vi "TWM Client Cmd Set Measurement.vi"(6 "Trigger":T1, 7 "end of packet key":string="TWM:command:EndOfPacket", 8 "error in":errorcluster, 9 "processing":T2, 10 "meas":T3, 11 "handle":i32) -> (0 "error out":errorcluster, 3 "handle out":i32)   [LabVIEW 2020, in "TWM Client.lvlib"]
doc: "Write Set measurement command packet to TWM server. Sets measurement configuration and processing configuration. The item \"valid?\" of the cluster(s) must be set to \"True\" to send the setup."
uses:
  TWM Client.lvlib
  TWM Client Meas Setup.ctl
  TWM Client Processing Setup.ctl
  TWM Client Meas Setup Trig.ctl
  I64.vi
  EXT.vi
  1D EXT.vi
  String.vi
  1D String.vi
  infolib.lvlib
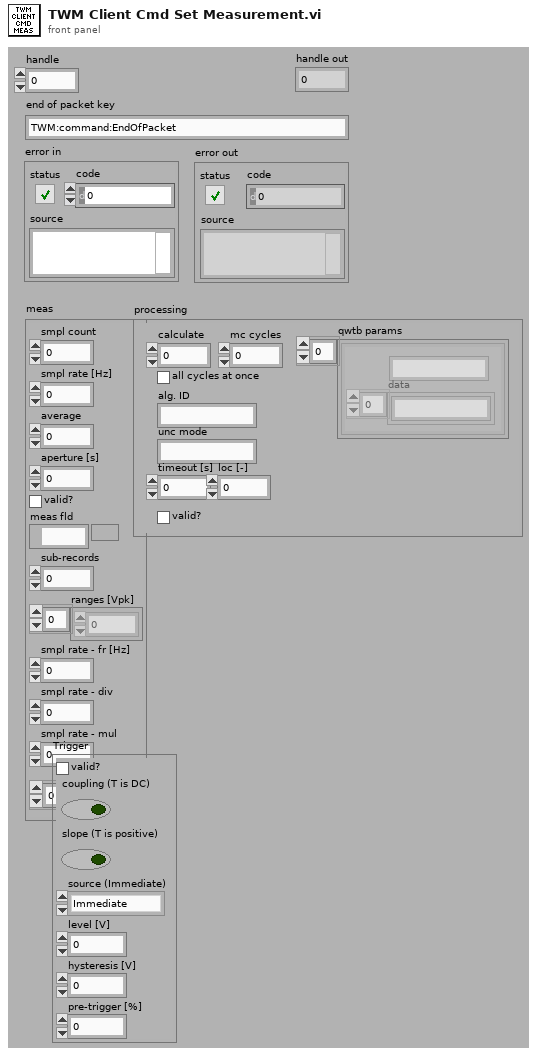
[diagram p1: front panel]
types:
  T1 = typedef "TWM Client.lvlib/TWM Client Meas Setup Trig.ctl" = cluster{"valid?":bool, "coupling (T is DC)":bool, "slope (T is positive)":bool, "source (Immediate)":enum16{"Immediate", "Level", "External"}, "level [V]":dbl, "hysteresis [V]":dbl, "pre-trigger [%]":dbl}
  T2 = typedef "TWM Client.lvlib/TWM Client Processing Setup.ctl" = cluster{"calculate":i32, "all cycles at once":bool, "alg. ID":string, "unc mode":string, "mc cycles":i32, "timeout [s]":dbl, "loc [-]":dbl, "valid?":bool, "qwtb params":cluster{"name":string, "data":string[]}[]}
  T3 = typedef "TWM Client.lvlib/TWM Client Meas Setup.ctl" = cluster{"smpl count":i32, "smpl rate [Hz]":dbl, "average":i32, "aperture [s]":dbl, "valid?":bool, "meas fld":path, "sub-records":i32, "ranges [Vpk]":dbl[], "smpl rate - fr [Hz]":dbl, "smpl rate - div":dbl, "smpl rate - mul":dbl, "offsets [V]":dbl[]}
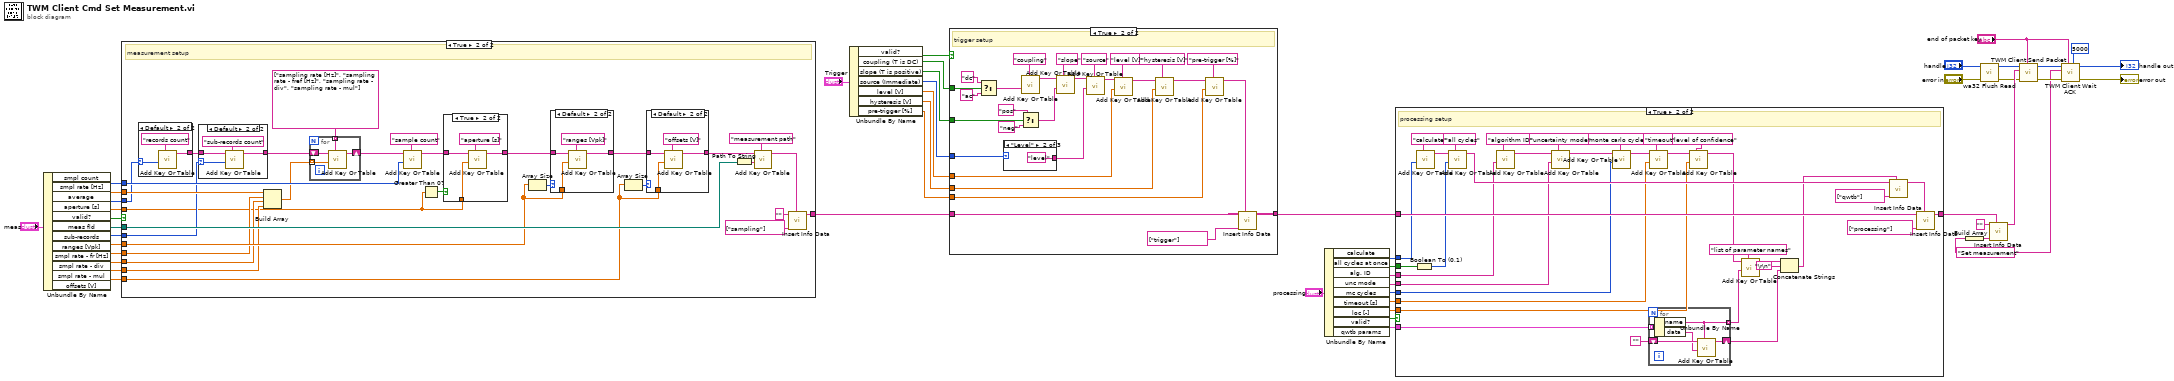
[diagram p0: block diagram]
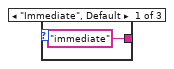
[diagram p3: hidden frame]
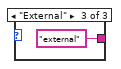
[diagram p4: hidden frame]
diagram:
  w21 = "Set measurement" ("section name")
  n1 = Unbundle By Name("meas") -> ("smpl count"=w45:i32, "smpl rate [Hz]"=w46:dbl, "average"=w47:i32, "aperture [s]"=w44:dbl, "valid?"=w43:bool, "meas fld"=w28:path, "sub-records"=w20:i32, "ranges [Vpk]"=w19:dbl[], "smpl rate - fr [Hz]"=w18:dbl, "smpl rate - div"=w17:dbl, "smpl rate - mul"=w16:dbl, "offsets [V]"=w1:dbl[])
  n2 = case shown="True" w43 {
    tunnel: [_ w78] -> w5
    tunnel: w47 -> [_ w63]
    tunnel: w46 -> [_ w74]
    tunnel: w45 -> [_ w73]
    tunnel: w44 -> [_ w53]
    tunnel: w28 -> [_ w68]
    tunnel: w20 -> [_ w64]
    tunnel: w19 -> [_ w60]
    tunnel: w18 -> [_ w57]
    tunnel: w17 -> [_ w56]
    tunnel: w16 -> [_ w55]
    tunnel: w1 -> [_ w49]
    frame False {
    }
    frame True {
      # "measurement setup"
      n3 = case shown="Default" w63 {
        selector: w63 -> [_ w98]
        tunnel: [_ w99] -> w66
        frame 0 {
        }
        frame Default {
          n4 = call-poly "Add Key Or Table.vi"("key description"="records count", "numeric"=w98) -> ("info data out"=w99:string)  [unwired: 8 in, 1 out]
        }
      }
      n5 = case shown="Default" w64 {
        selector: w64 -> [_ w102]
        tunnel: w66 -> [w101 w104]
        tunnel: [w101 w103] -> w65
        frame 0 {
        }
        frame Default {
          n6 = call-poly "Add Key Or Table.vi"("key description"="sub-records count", "numeric"=w102, "info data"=w104) -> ("info data out"=w103:string)  [unwired: 7 in, 1 out]
        }
      }
      n7 = Build Array(w74, w57, w56, w55) -> (w58:dbl[])
      n8 = for {
        tunnel: w58 -> [w91] mode=indexing
        tunnel: string[] ["sampling rate [Hz]", "sampling rate - fref [Hz]", "sampling rate - div", "sampling rate - mul"] -> [w89] mode=indexing
        shift-right: [w92] -> w76
        shift-left: w65 -> [w90]
        n9 = call-poly "Add Key Or Table.vi"("key description"=w89, "numeric"=w91, "info data"=w90) -> ("info data out"=w92:string)  [unwired: 7 in, 1 out]
      }
      n10 = call-poly "Add Key Or Table.vi"("key description"="sample count", "numeric"=w73, "info data"=w76) -> ("info data out"=w75:string)  [unwired: 7 in, 1 out]
      n11 = Greater Than 0?(x=w53) -> (x > 0?=w54:bool)
      n12 = case shown="True" w54 {
        tunnel: w75 -> [w84 w88]
        tunnel: w53 -> [_ w87]
        tunnel: [w84 w85] -> w62
        frame False {
        }
        frame True {
          n13 = call-poly "Add Key Or Table.vi"("key description"="aperture [s]", "numeric"=w87, "info data"=w88) -> ("info data out"=w85:string)  [unwired: 7 in, 1 out]
        }
      }
      n14 = Array Size(array=w60) -> (size(s)=w61:i32)
      n15 = case shown="Default" w61 {
        tunnel: w62 -> [w93 w96]
        tunnel: [w93 w95] -> w51
        tunnel: w60 -> [_ w94]
        frame 0 {
          # "do not send\nwhen array empty"
        }
        frame Default {
          n16 = call-poly "Add Key Or Table.vi"("key description"="ranges [Vpk]", "numeric"=w94, "info data"=w96) -> ("info data out"=w95:string)  [unwired: 7 in, 1 out]
        }
      }
      n17 = Array Size(array=w49) -> (size(s)=w52:i32)
      n18 = case shown="Default" w52 {
        tunnel: w51 -> [w79 w82]
        tunnel: [w79 w81] -> w50
        tunnel: w49 -> [_ w80]
        frame 0 {
          # "do not send\nwhen array empty"
        }
        frame Default {
          n19 = call-poly "Add Key Or Table.vi"("key description"="offsets [V]", "numeric"=w80, "info data"=w82) -> ("info data out"=w81:string)  [unwired: 7 in, 1 out]
        }
      }
      n20 = Path To String(path=w68) -> (string=w67:string)
      n21 = call-poly "Add Key Or Table.vi"("key description"="measurement path", "string"=w67, "info data"=w50) -> ("info data out"=w69:string)  [unwired: 7 in, 1 out]
      n22 = call "Insert Info Data.vi"("info data to insert"=w69, "sections"=string[] ["sampling"], "info data"="") -> ("info data out"=w78:string)  [unwired: 7 in, 1 out]
    }
  }
  n23 = Unbundle By Name("Trigger") -> ("valid?"=w10:bool, "coupling (T is DC)"=w9:bool, "slope (T is positive)"=w8:bool, "source (Immediate)"=w7:enum16{"Immediate", "Level", "External"}, "level [V]"=w6:dbl, "hysteresis [V]"=w3:dbl, "pre-trigger [%]"=w2:dbl)
  n24 = case shown="True" w10 {
    tunnel: w9 -> [_ w133]
    tunnel: w8 -> [_ w126]
    tunnel: w7 -> [_ w121]
    tunnel: w6 -> [_ w117]
    tunnel: w5 -> [w106 w116]
    tunnel: [w106 w115] -> w4
    tunnel: w3 -> [_ w108]
    tunnel: w2 -> [_ w107]
    frame False {
    }
    frame True {
      # "trigger setup"
      n25 = Select(t="dc" ("key description"), s=w133, f="ac" ("key description")) -> (s? t:f=w130:string)
      n26 = case shown="\"Level\"" w121 {
        tunnel: ["immediate" ("key description") "level" ("key description") "external" ("key description")] -> w120
        frame "Immediate", Default {
        }
        frame "Level" {
        }
        frame "External" {
        }
      }
      n27 = Select(t="pos" ("key description"), s=w126, f="neg" ("key description")) -> (s? t:f=w128:string)
      n28 = call-poly "Add Key Or Table.vi"("key description"="coupling", "string"=w130) -> ("info data out"=w125:string)  [unwired: 8 in, 1 out]
      n29 = call-poly "Add Key Or Table.vi"("key description"="slope", "string"=w128, "info data"=w125) -> ("info data out"=w123:string)  [unwired: 7 in, 1 out]
      n30 = call-poly "Add Key Or Table.vi"("key description"="source", "string"=w120, "info data"=w123) -> ("info data out"=w119:string)  [unwired: 7 in, 1 out]
      n31 = call-poly "Add Key Or Table.vi"("key description"="level [V]", "numeric"=w117, "info data"=w119) -> ("info data out"=w112:string)  [unwired: 7 in, 1 out]
      n32 = call-poly "Add Key Or Table.vi"("key description"="hysteresis [V]", "numeric"=w108, "info data"=w112) -> ("info data out"=w110:string)  [unwired: 7 in, 1 out]
      n33 = call-poly "Add Key Or Table.vi"("key description"="pre-trigger [%]", "numeric"=w107, "info data"=w110) -> ("info data out"=w109:string)  [unwired: 7 in, 1 out]
      n34 = call "Insert Info Data.vi"("info data to insert"=w109, "sections"=string[] ["trigger"], "info data"=w116) -> ("info data out"=w115:string)  [unwired: 7 in, 1 out]
    }
  }
  n35 = Unbundle By Name("processing") -> ("calculate"=w41:i32, "all cycles at once"=w40:bool, "alg. ID"=w39:string, "unc mode"=w38:string, "mc cycles"=w37:i32, "timeout [s]"=w36:dbl, "loc [-]"=w35:dbl, "valid?"=w34:bool, "qwtb params"=w29:cluster{"name":string, "data":string[]}[])
  n36 = case shown="True" w34 {
    tunnel: w4 -> [w138 w173]
    tunnel: w41 -> [_ w156]
    tunnel: w40 -> [_ w155]
    tunnel: w39 -> [_ w153]
    tunnel: w38 -> [_ w152]
    tunnel: w37 -> [_ w151]
    tunnel: w36 -> [_ w150]
    tunnel: w35 -> [_ w149]
    tunnel: [w138 w148] -> w33
    tunnel: w29 -> [_ w146]
    frame False {
    }
    frame True {
      # "processing setup"
      n37 = Boolean To (0,1)(Boolean=w155) -> (0, 1=w154:i16)
      n38 = call-poly "Add Key Or Table.vi"("key description"="calculate", "numeric"=w156) -> ("info data out"=w170:string)  [unwired: 8 in, 1 out]
      n39 = call-poly "Add Key Or Table.vi"("key description"="all cycles", "numeric"=w154, "info data"=w170) -> ("info data out"=w157:string)  [unwired: 7 in, 1 out]
      n40 = call-poly "Add Key Or Table.vi"("key description"="algorithm ID", "string"=w153) -> ("info data out"=w171:string)  [unwired: 8 in, 1 out]
      n41 = call-poly "Add Key Or Table.vi"("key description"="uncertainty mode", "string"=w152, "info data"=w171) -> ("info data out"=w161:string)  [unwired: 7 in, 1 out]
      n42 = call-poly "Add Key Or Table.vi"("key description"="monte carlo cycles", "numeric"=w151, "info data"=w161) -> ("info data out"=w163:string)  [unwired: 7 in, 1 out]
      n43 = for {
        tunnel: w146 -> [w178] mode=indexing
        tunnel: [w177] -> w140 mode=indexing
        shift-right: [w175] -> w139
        shift-left: "" -> [w176]
        n44 = Unbundle By Name(w178) -> ("name"=w177:string, "data"=w174:string[])
        n45 = call-poly "Add Key Or Table.vi"("key description"=w177, "string"=w174, "info data"=w176) -> ("info data out"=w175:string)  [unwired: 7 in, 1 out]
      }
      n46 = call-poly "Add Key Or Table.vi"("key description"="timeout", "numeric"=w150, "info data"=w163) -> ("info data out"=w160:string)  [unwired: 7 in, 1 out]
      n47 = call-poly "Add Key Or Table.vi"("key description"="level of confidence", "numeric"=w149, "info data"=w160) -> ("info data out"=w142:string)  [unwired: 7 in, 1 out]
      n48 = call-poly "Add Key Or Table.vi"("key description"="list of parameter names", "string"=w140, "info data"=w142) -> ("info data out"=w144:string)  [unwired: 7 in, 1 out]
      n49 = Concatenate Strings(w144, "\r\n", w139) -> (w141:string)
      n50 = call "Insert Info Data.vi"("info data to insert"=w141, "sections"=string[] ["qwtb"], "info data"=w157) -> ("info data out"=w158:string)  [unwired: 7 in, 1 out]
      n51 = call "Insert Info Data.vi"("info data to insert"=w158, "sections"=string[] ["processing"], "info data"=w173) -> ("info data out"=w148:string)  [unwired: 7 in, 1 out]
    }
  }
  n52 = Build Array(w21) -> (w31:string[])
  n53 = call "wa32 Flush Read.vi"("error in"="error in", "handle"="handle") -> ("error out"=w14:errorcluster, "handle out"=w13:i32)  [unwired: 7 in, 1 out]
  n54 = call "Insert Info Data.vi"("info data to insert"=w33, "sections"=w31, "info data"="") -> ("info data out"=w32:string)  [unwired: 7 in, 1 out]
  n55 = call "TWM Client Send Packet.vi"("end of packet key"="end of packet key", "error in"=w14, "command string"=w32, "handle"=w13) -> ("error out"=w27:errorcluster, "handle out"=w26:i32)  [unwired: 6 in]
  n56 = call "TWM Client Wait ACK.vi"("timeout [ms] (3000)"=5000 ("timeout [ms] (1000)"), "key string"="end of packet key", "error in"=w27, "command header"=w21, "handle"=w26) -> ("error out"=→"error out":errorcluster, "handle out"=→"handle out":i32)  [unwired: 5 in]
